vi "离线读数据.vi"(7 "通道数":i32, 8 "错误输入":errorcluster caption="输出簇", 9 "读取字节数":u32, 10 "读取位置":i32, 11 "文件句柄":i32) -> (0 "错误输出":errorcluster, 1 "实际字节数":u32, 2 "AD原码":u16[][](array[numeric]), 3 "文件句柄出":i32, 4 "AD物理值":dbl[][](array[numeric]))   [LabVIEW 2011]
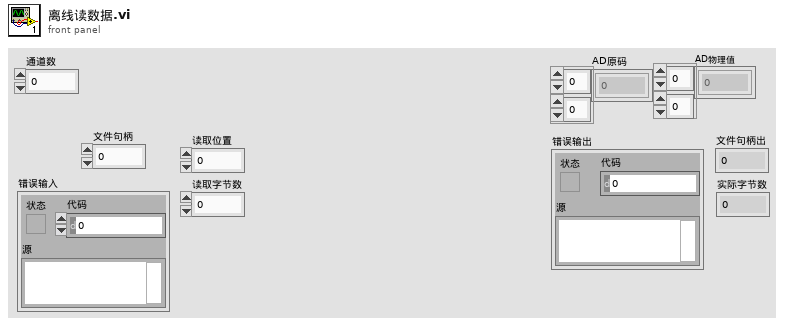
[diagram p1: front panel]
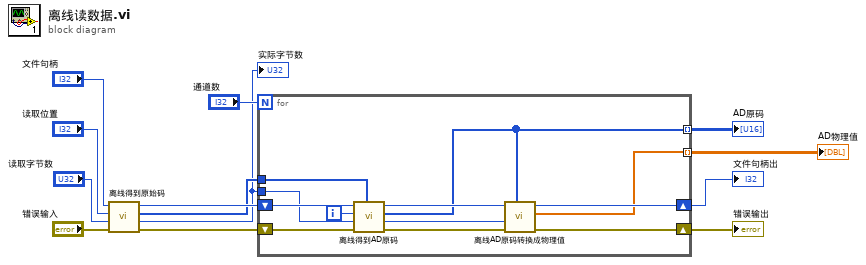
[diagram p0: block diagram]
diagram:
  n1 = call "离线得到原始码.vi"("错误输入"="错误输入", "读取字节数"="读取字节数", "读取位置"="读取位置", "文件句柄"="文件句柄") -> ("错误输出"=w11:errorcluster, "实际字节数"=w2:u32, "原始码"=w12:u8[], "文件句柄出"=w13:i32)  [unwired: 4 in]
  "实际字节数" <- w2
  n2 = for {
    N: "通道数" -> [_]
    tunnel: w2 -> [w24]
    shift-right: [w19] -> w7
    shift-left: w13 -> [w25]
    tunnel: [w15] -> w6 mode=indexing
    tunnel: w12 -> [w22]
    shift-right: [w17] -> w4
    shift-left: w11 -> [w21]
    tunnel: [w16] -> w1 mode=indexing
    i -> [w23]
    n3 = call "离线得到AD原码.vi"("原始码"=w22, "错误输入"=w21, "原始码字节数"=w24, "通道索引"=w23, "文件句柄"=w25) -> ("错误输出"=w18:errorcluster, "数据个数"=w14:u32, "AD原码"=w15:u16[], "文件句柄出"=w20:i32)  [unwired: 3 in]
    n4 = call "离线AD原码转换成物理值 .vi"("原始码"=w15, "错误输入"=w18, "AD数据个数"=w14, "文件句柄"=w20) -> ("错误输出"=w17:errorcluster, "AD物理值"=w16:dbl[], "文件句柄出"=w19:i32)  [unwired: 5 in]
  }
  "文件句柄出" <- w7
  "AD原码" <- w6
  "错误输出" <- w4
  "AD物理值" <- w1
